vi "ProcAndStates.vi"(0 "spreadsheet string":string=" Инициализация\r\nНачало\r\nВосстановлениеУправления\r\nНачалоРаботы\r\n ОстановВсехПроцессовИстартПроцИнициализация\r\nНачало\r\n КонтрольДостоверности\r\nНачало\r\nОстановПроцессов\r\nСообК_ГУИ_НЕТ_ДОСТОВЕРНОСТИ\r\nНарушениеСвязи\r\n КонтрольДостоверностиОткрытияЗатвораВакуумного\r\nНачало\r\nСменаСостоянияВКЛ\r\nСменаСостоянияВЫКЛ\r\nТрафикПауза\r\nНарушениеСвязи\r\n КонтрольДостоверностиОткрЗатВакуумного\r\nНачало\r\nСообК_ГУИ_ЕСТЬ_ДОСТОВЕРНОСТЬ\r\nОжиданиеНедостоверности\r\nСообК_ГУИ_НЕТ_ДОСТОВЕРНОСТИ\r\nОжиданиеЕстьДостоверность\r\nНарушениеСвязи\r\n КонтрольДостоверностиЗакрЗатВакуумного\r\nНачало\r\nСообК_ГУИ_ЕСТЬ_ДОСТОВЕРНОСТЬ\r\nОжиданиеНедостоверности\r\nСообК_ГУИ_НЕТ_ДОСТОВЕРНОСТИ\r\nОжиданиеЕстьДостоверность\r\nНарушениеСвязи\r\n КонтрольДостоверностиСостоянияСапуна\r\nНачало\r\nСообК_ГУИ_ЕСТЬ_ДОСТОВЕРНОСТЬ\r\nОжиданиеНедостоверности\r\nСообК_ГУИ_НЕТ_ДОСТОВЕРНОСТИ\r\nОжиданиеЕстьДостоверность\r\nНарушениеСвязи\r\n КонтрольДостоверностиСостоянияУстройстваПлавПуска\r\nНачало\r\nСообК_ГУИ_ЕСТЬ_ДОСТОВЕРНОСТЬ\r\nОжиданиеНедостоверности\r\nСообК_ГУИ_НЕТ_ДОСТОВЕРНОСТИ\r\nОжиданиеЕстьДостоверность\r\nНарушениеСвязи\r\n КонтрольДостоверностиСостоянияПитанияВакуумногоНасоса\r\nНачало\r\nСообК_ГУИ_ЕСТЬ_ДОСТОВЕРНОСТЬ\r\nОжиданиеНедостоверности\r\nСообК_ГУИ_НЕТ_ДОСТОВЕРНОСТИ\r\nОжиданиеЕстьДостоверность\r\nНарушениеСвязи\r\n КонтрольДостоверностиСостоянияПитанияВентилятора\r\nНачало\r\nСообК_ГУИ_ЕСТЬ_ДОСТОВЕРНОСТЬ\r\nОжиданиеНедостоверности\r\nСообК_ГУИ_НЕТ_ДОСТОВЕРНОСТИ\r\nОжиданиеЕстьДостоверность\r\nНарушениеСвязи\r\n КонтрольДостоверностиСостоянияПитанияРегТемпературы\r\nНачало\r\nСообК_ГУИ_ЕСТЬ_ДОСТОВЕРНОСТЬ\r\nОжиданиеНедостоверности\r\nСообК_ГУИ_НЕТ_ДОСТОВЕРНОСТИ\r\nОжиданиеЕстьДостоверность\r\nНарушениеСвязи\r\n КонтрольДостоверностиСостоянияПитанияРегУровня\r\nНачало\r\nСообК_ГУИ_ЕСТЬ_ДОСТОВЕРНОСТЬ\r\nОжиданиеНедостоверности\r\nСообК_ГУИ_НЕТ_ДОСТОВЕРНОСТИ\r\nОжиданиеЕстьДостоверность\r\nНарушениеСвязи\r\n КонтрольДостоверностиУровняВодыМинимум\r\nНачало\r\nСообК_ГУИ_ЕСТЬ_ДОСТОВЕРНОСТЬ\r\nОжиданиеНедостоверности\r\nСообК_ГУИ_НЕТ_ДОСТОВЕРНОСТИ\r\nОжиданиеЕстьДостоверность\r\nНарушениеСвязи\r\n КонтрольДостоверностиУровняВодыМаксимум\r\nНачало\r\nСообК_ГУИ_ЕСТЬ_ДОСТОВЕРНОСТЬ\r\nОжиданиеНедостоверности\r\nСообК_ГУИ_НЕТ_ДОСТОВЕРНОСТИ\r\nОжиданиеЕстьДостоверность\r\nНарушениеСвязи\r\n КонтрольДостоверностиСостоянияПитанияНасОхлаждения\r\nНачало\r\nСообК_ГУИ_ЕСТЬ_ДОСТОВЕРНОСТЬ\r\nОжиданиеНедостоверности\r\nСообК_ГУИ_НЕТ_ДОСТОВЕРНОСТИ\r\nОжиданиеЕстьДостоверность\r\nНарушениеСвязи\r\n ЧтениеФактПараметров_с_Датчиков\r\nНачало\r\n РЕГУЛЯТОР_ТРАФИКА\r\nНачало\r\n ЧтениеКольцевогоБуфера\r\nНачало\r\nКонтрольВыполненияК\r\nКонтрольИзмененияНП\r\nНекорректноеСобытие\r\nНарушениеСвязи\r\n ОбработкаКомандИзмененияНП_от_ГУИ\r\nАнализ\r\nПодтверждениеИзмененияНП\r\nНекорректноеСобытие\r\nНарушениеСвязи\r\n ОбработкаКомандУправления_от_ГУИ\r\nАнализ\r\nНекорректноеСобытие\r\nПередачаСообщенияСПараметромГУИ\r\nНарушениеСвязи\r\n КонтрольИзменения_ФП_P_ВбакеКомпрессора\r\nНачало\r\nКонтрольИзменения\r\nСообщОбИзменении\r\nТрафикПауза\r\nНарушениеСвязи\r\n КонтрольИзменения_ФП_P_Впатрубке\r\nНачало\r\nКонтрольИзменения\r\nСообщОбИзменении\r\nТрафикПауза\r\nНарушениеСвязи\r\n КонтрольИзменения_ФП_T_Врубашке\r\nНачало\r\nКонтрольИзменения\r\nСообщОбИзменении\r\nТрафикПауза\r\nНарушениеСвязи\r\n КонтрольИзменения_ФП_T_Вбаке\r\nНачало\r\nКонтрольИзменения\r\nСообщОбИзменении\r\nТрафикПауза\r\nНарушениеСвязи\r\n КонтрольИзменения_ФП_P_ВтрубеСидер\r\nНачало\r\nКонтрольИзменения\r\nСообщОбИзменении\r\nТрафикПауза\r\nНарушениеСвязи\r\n КонтрольВеличиныОткачкиВауумнойТрубыСидеростата\r\nНачало\r\nАнализОткачки\r\n КонтрольГотовностиВакуума_в_Вакуумной_Трубе\r\nНачало\r\nДавлениеНормальное\r\nДавлениеВысокое\r\nЗадержка\r\nНарушениеСвязи\r\n КонтрольУровняВодыБакаОхлаждения\r\nНачало\r\nНизкийУровеньВоды\r\nВысокийУровеньВоды\r\nУровеньВодыВнорме\r\nЗадержка\r\nНарушениеСвязи\r\n КонтрольТемпературыВодыБакаОхлаждения\r\nНачало\r\nНизкаяТемператураВоды\r\nВысокаяТемператураВоды\r\nТемператураВнорме\r\nЗадержка\r\nНарушениеСвязи\r\n КонтрольТемпературыРубашкиОхлаждения\r\nНачало\r\nНизкаяТемператураВоды\r\nВысокаяТемператураВоды\r\nТемператураВнорме\r\nЗадержка\r\nНарушениеСвязи\r\n КонтрольДавленияВбакеКомпрессора\r\nНачало\r\nНизкоеДавление\r\nДавлениеВнорме\r\nЗадержка\r\nНарушениеСвязи\r\n ВКЛ_ПИТ_ВЕНТИЛЯТОР\r\nНачало\r\nКонтрольВключения\r\nПередачаСообщения\r\nОшибка\r\nНарушениеСвязи\r\n ВЫК_ПИТ_ВЕНТИЛЯТОР\r\nНачало\r\nКонтрольВыключения\r\nПередачаСообщения\r\nОшибка\r\nНарушениеСвязи\r\n КонтрольСостоянияПитанияВентилятора\r\nНачало\r\nСменаСостоянияВКЛ\r\nСменаСостоянияВЫКЛ\r\nНарушениеСвязи\r\n КонтрольСпонтанногоВыключенияВентилятора\r\nКонтроль\r\nОшибка\r\nНарушениеСвязи\r\n КонтрольСпонтанногоВключенияВентилятора\r\nКонтроль\r\nОшибка\r\nНарушениеСвязи\r\n КонтрольСостоянияЗатвораВакуумного\r\nНачало\r\nСменаСостоянияСреднего\r\nСменаСостоянияЗакрытия\r\nСменаСостоянияОткрытия\r\nСменаСостоянияОшибки\r\nНарушениеСвязи\r\n ОТКР_ЗАТВОР_ВАК\r\nНачало\r\nКонтроль\r\nПередачаСообщения\r\nОшибка\r\nНарушениеСвязи\r\n ЗАКР_ЗАТВОР_ВАК\r\nНачало\r\nКонтроль\r\nПередачаСообщения\r\nОшибка\r\nНарушениеСвязи\r\n КонтрольСпонтанногоЗакрытияЗатвораВакуумного\r\nКонтрольЗакрытия\r\nОшибка\r\nНарушениеСвязи\r\n КонтрольСпонтанногоОткрытияЗатвораВакуумного\r\nКонтроль\r\nОшибка\r\nНарушениеСвязи\r\n ОТКР_САПУН\r\nНачало\r\nКонтрольОткрытия\r\nПередачаСообщения\r\nОшибка\r\nНарушениеСвязи\r\n ЗАКР_САПУН\r\nНачало\r\nКонтрольЗакрытия\r\nПередачаСообщения\r\nОшибка\r\nНарушениеСвязи\r\n КонтрольСостоянияПитанияСапуна\r\nНачало\r\nСменаСостоянияВКЛ\r\nСменаСостоянияВЫКЛ\r\nНарушениеСвязи\r\n КонтрольСпонтанногоЗакрытияСапуна\r\nКонтрольЗакрытия\r\nОшибка\r\nНарушениеСвязи\r\n КонтрольСпонтанногоОткрытияСапуна\r\nКонтроль\r\nОшибка\r\nНарушениеСвязи\r\n ВКЛ_ПИТ_ВАК_НАСОСА\r\nНачало\r\nКонтрольВключения\r\nПередачаСообщения\r\nОшибка\r\nНарушениеСвязи\r\n ВЫК_ПИТ_ВАК_НАСОСА\r\nНачало\r\nКонтрольВыключения\r\nОшибка\r\nНарушениеСвязи\r\nПередачаСообщения\r\n КонтрольСостоянияПитанияВакуумногоНасоса\r\nНачало\r\nСменаСостоянияВКЛ\r\nСменаСостоянияВЫКЛ\r\nНарушениеСвязи\r\n КонтрольСпонтанногоВыключенияВакНасоса\r\nКонтроль\r\nОшибка\r\nНарушениеСвязи\r\n КонтрольСпонтанногоВключенияВакНасоса\r\nКонтроль\r\nОшибка\r\nНарушениеСвязи\r\n ВКЛ_ПИТ_РЕГ_Т\r\nНачало\r\nКонтрольВключения\r\nПередачаСообщения\r\nОшибка\r\nНарушениеСвязи\r\n ВЫК_ПИТ_РЕГ_Т\r\nНачало\r\nКонтрольВыключения\r\nПередачаСообщения\r\nОшибка\r\nНарушениеСвязи\r\n КонтрольСостоянияПитанияРЕГ_Т\r\nНачало\r\nСменаСостоянияВКЛ\r\nСменаСостоянияВЫКЛ\r\nНарушениеСвязи\r\n КонтрольСпонтанногоВыключенияРЕГ_Т\r\nКонтроль\r\nОшибка\r\nНарушениеСвязи\r\n КонтрольСпонтанногоВключенияРЕГ_Т\r\nКонтроль\r\nОшибка\r\nНарушениеСвязи\r\n ВКЛ_ПИТ_РЕГ_УР\r\nНачало\r\nКонтроль\r\nПередачаСообщения\r\nОшибка\r\nНарушениеСвязи\r\n ВЫК_ПИТ_РЕГ_УР\r\nНачало\r\nКонтроль\r\nПередачаСообщения\r\nОшибка\r\nНарушениеСвязи\r\n КонтрольСостоянияПитанияРЕГ_УР\r\nНачало\r\nСменаСостоянияВКЛ\r\nСменаСостоянияВЫКЛ\r\nНарушениеСвязи\r\n КонтрольСпонтанногоВыключенияРЕГ_УР\r\nКонтроль\r\nОшибка\r\nНарушениеСвязи\r\n КонтрольСпонтанногоВключенияРЕГ_УР\r\nКонтроль\r\nОшибка\r\nНарушениеСвязи\r\n ВКЛ_ПИТ_НАС_ОХЛ\r\nНачало\r\nВключениеПитания\r\nКонтроль\r\nПередачаСообщения\r\nОшибка\r\nНарушениеСвязи\r\n ВЫК_ПИТ_НАС_ОХЛ\r\nНачало\r\nКонтроль\r\nПередачаСообщения\r\nОшибка\r\nНарушениеСвязи\r\n КонтрольСостоянияПитанияНАС_ОХЛ\r\nНачало\r\nСменаСостоянияВКЛ\r\nСменаСостоянияВЫКЛ\r\nНарушениеСвязи\r\n КонтрольСпонтанногоВыключенияНасосаОхлаждения\r\nКонтроль\r\nОшибка\r\nНарушениеСвязи\r\n КонтрольСпонтанногоВключенияНасосаОхлаждения\r\nКонтроль\r\nОшибка\r\nНарушениеСвязи\r\n ВКЛ_УСТР_ПЛАВ_ПУСКА\r\nНачало\r\nКонтроль\r\nПередачаСообщения\r\nОшибка\r\nНарушениеСвязи\r\n ВЫК_УСТР_ПЛАВ_ПУСКА\r\nНачало\r\nКонтрольВыключения\r\nПередачаСообщения\r\nОшибка\r\nНарушениеСвязи\r\n КонтрольСостоянияПитанияПЛАВ_ПУСКА\r\nНачало\r\nСменаСостоянияВКЛ\r\nСменаСостоянияВЫКЛ\r\nНарушениеСвязи\r\n КонтрольСпонтанногоВыключенияПлавнПуска\r\nКонтроль\r\nОшибка\r\nНарушениеСвязи\r\n КонтрольСпонтанногоВключенияПлавнПуска\r\nКонтроль\r\nОшибка\r\nНарушениеСвязи\r\n ВКЛ_ВАКУУМИРОВАНИЕ_ТРУБЫ\r\nНачало\r\nПроверкаНеобходимостиВакуумирования\r\nПередачаСообщения\r\nКонтрольВключенияВакПодсистемы\r\nЗапоминаемДавлениеВвакуумнойТрубе\r\nКонтрольТемпературыРубашки\r\nКонтрольРаботыОборудования\r\nКонтрольДавления\r\nСообщениеОКонцеВакуумирования\r\nПаузаНаРазвакуумированиеТрубы\r\nПаузаНаОткачкуВвакуумнойТрубе\r\nПроверкаУменьшенияДавленияВпатрубке\r\nОткачкаОтсутствует\r\nВыключениеВакуумнойПодсистемы\r\nСообщениеОбОтказеВакуумирования\r\nНарушениеСвязи\r\n ВЫК_ВАКУУМИРОВАНИЕ_ТРУБЫ\r\nНачало\r\nПередачаСообщения\r\nВыключениеВакуумнойПодсистемы\r\nНарушениеСвязи\r\n ВКЛ_ВАКУУМНУЮ_ПОДСИСТЕМУ\r\nНачало\r\nВключениеПитанияРегУровня\r\nКонтрольВключенияПитРегУр\r\nКонтрольГотовностиУровняВодыБО\r\nВключениеРегТ\r\nКонтрольВключенияРегТ\r\nКонтрольПревышенияТемпературыВодыБО\r\nКонтрольГотовностиТемпературыВодыБО\r\nВключаемВентилятор\r\nКонтрольВключенияВентилятора\r\nКонтрольВключенияПитанияНасосаОхлаждения\r\nКонтрольЗакрытияЗатвораВакуумного\r\nКонтрольОткрытияСапуна\r\nКонтрольТемпературыРубашки\r\nПодачаПитанияНаВакуумныйНасос\r\nКонтрольПитанияВакуумногоНасоса\r\nВключениеУстройстваПлавногоПуска\r\nКонтрольВлюченияПлавногоПуска\r\nТаймаутПередЗакрытиемСапуна\r\nЗакрытиеСапуна\r\nКонтрольЗакрытияСапуна\r\nЗапоминаемДавлениеВпатрубке\r\nКонтрольДавления\r\nПаузаНаОткачкуВпатрубке\r\nПроверкаУменьшенияДавленияВпатрубке\r\nКонтрольОткрытияЗВ\r\nОшибка\r\nВыключениеПоОшибке\r\nСообщениеОбОтказеВакуумирования\r\nНарушениеСвязи\r\n ВЫК_ВАКУУМНУЮ_ПОДСИСТЕМУ\r\nНачало\r\nКонтрольЗакрытияЗатвораВакуумного\r\nКонтрольОткрытияСапуна\r\nТаймаутПередВыключениемПитанияВакуумногоНасоса\r\nВыключаемУППВакуумногоНасоса\r\nКонтрольВыключенияПитанияУППВакуумногоНасоса\r\nКонтрольВыключенияПитанияВакуумногоНасоса\r\nКонтрольВыключенияНасосаОхлаждения\r\nКонтрольВыключенияВентилятора\r\nСообщениеОбОтказеВыклВакСистемы\r\nНарушениеСвязи\r\n") -> (1 "PROCESSES":string[](array[string])=["Инициализация", "ОстановВсехПроцессовИстартПроцИнициализация", "КонтрольДостоверности", "КонтрольДостоверностиОткрытияЗатвораВакуумного", "КонтрольДостоверностиОткрЗатВакуумного", "КонтрольДостоверностиЗакрЗатВакуумного", "КонтрольДостоверностиСостоянияСапуна", "КонтрольДостоверностиСостоянияУстройстваПлавПуска", "КонтрольДостоверностиСостоянияПитанияВакуумногоНасоса", "КонтрольДостоверностиСостоянияПитанияВентилятора", "КонтрольДостоверностиСостоянияПитанияРегТемпературы", "КонтрольДостоверностиСостоянияПитанияРегУровня", "КонтрольДостоверностиУровняВодыМинимум", "КонтрольДостоверностиУровняВодыМаксимум", "КонтрольДостоверностиСостоянияПитанияНасОхлаждения", "ЧтениеФактПараметров_с_Датчиков", "РЕГУЛЯТОР_ТРАФИКА", "ЧтениеКольцевогоБуфера", "ОбработкаКомандИзмененияНП_от_ГУИ", "ОбработкаКомандУправления_от_ГУИ", "КонтрольИзменения_ФП_P_ВбакеКомпрессора", "КонтрольИзменения_ФП_P_Впатрубке", "КонтрольИзменения_ФП_T_Врубашке", "КонтрольИзменения_ФП_T_Вбаке", "КонтрольИзменения_ФП_P_ВтрубеСидер", "КонтрольВеличиныОткачкиВауумнойТрубыСидеростата", "КонтрольГотовностиВакуума_в_Вакуумной_Трубе", "КонтрольУровняВодыБакаОхлаждения", "КонтрольТемпературыВодыБакаОхлаждения", "КонтрольТемпературыРубашкиОхлаждения", "КонтрольДавленияВбакеКомпрессора", "ВКЛ_ПИТ_ВЕНТИЛЯТОР", "ВЫК_ПИТ_ВЕНТИЛЯТОР", "КонтрольСостоянияПитанияВентилятора", "КонтрольСпонтанногоВыключенияВентилятора", "КонтрольСпонтанногоВключенияВентилятора", "КонтрольСостоянияЗатвораВакуумного", "ОТКР_ЗАТВОР_ВАК", "ЗАКР_ЗАТВОР_ВАК", "КонтрольСпонтанногоЗакрытияЗатвораВакуумного", "КонтрольСпонтанногоОткрытияЗатвораВакуумного", "ОТКР_САПУН", "ЗАКР_САПУН", "КонтрольСостоянияПитанияСапуна", "КонтрольСпонтанногоЗакрытияСапуна", "КонтрольСпонтанногоОткрытияСапуна", "ВКЛ_ПИТ_ВАК_НАСОСА", "ВЫК_ПИТ_ВАК_НАСОСА", "КонтрольСостоянияПитанияВакуумногоНасоса", "КонтрольСпонтанногоВыключенияВакНасоса", "КонтрольСпонтанногоВключенияВакНасоса", "ВКЛ_ПИТ_РЕГ_Т", "ВЫК_ПИТ_РЕГ_Т", "КонтрольСостоянияПитанияРЕГ_Т", "КонтрольСпонтанногоВыключенияРЕГ_Т", "КонтрольСпонтанногоВключенияРЕГ_Т", "ВКЛ_ПИТ_РЕГ_УР", "ВЫК_ПИТ_РЕГ_УР", "КонтрольСостоянияПитанияРЕГ_УР", "КонтрольСпонтанногоВыключенияРЕГ_УР", "КонтрольСпонтанногоВключенияРЕГ_УР", "ВКЛ_ПИТ_НАС_ОХЛ", "ВЫК_ПИТ_НАС_ОХЛ", "КонтрольСостоянияПитанияНАС_ОХЛ", "КонтрольСпонтанногоВыключенияНасосаОхлаждения", "КонтрольСпонтанногоВключенияНасосаОхлаждения", "ВКЛ_УСТР_ПЛАВ_ПУСКА", "ВЫК_УСТР_ПЛАВ_ПУСКА", "КонтрольСостоянияПитанияПЛАВ_ПУСКА", "КонтрольСпонтанногоВыключенияПлавнПуска", "КонтрольСпонтанногоВключенияПлавнПуска", "ВКЛ_ВАКУУМИРОВАНИЕ_ТРУБЫ", "ВЫК_ВАКУУМИРОВАНИЕ_ТРУБЫ", "ВКЛ_ВАКУУМНУЮ_ПОДСИСТЕМУ", "ВЫК_ВАКУУМНУЮ_ПОДСИСТЕМУ"], 2 "STATES":string[][](array[string]))   [LabVIEW 2012]
panel:
  out "size(s)":i32[](array[numeric])=[75, 0]
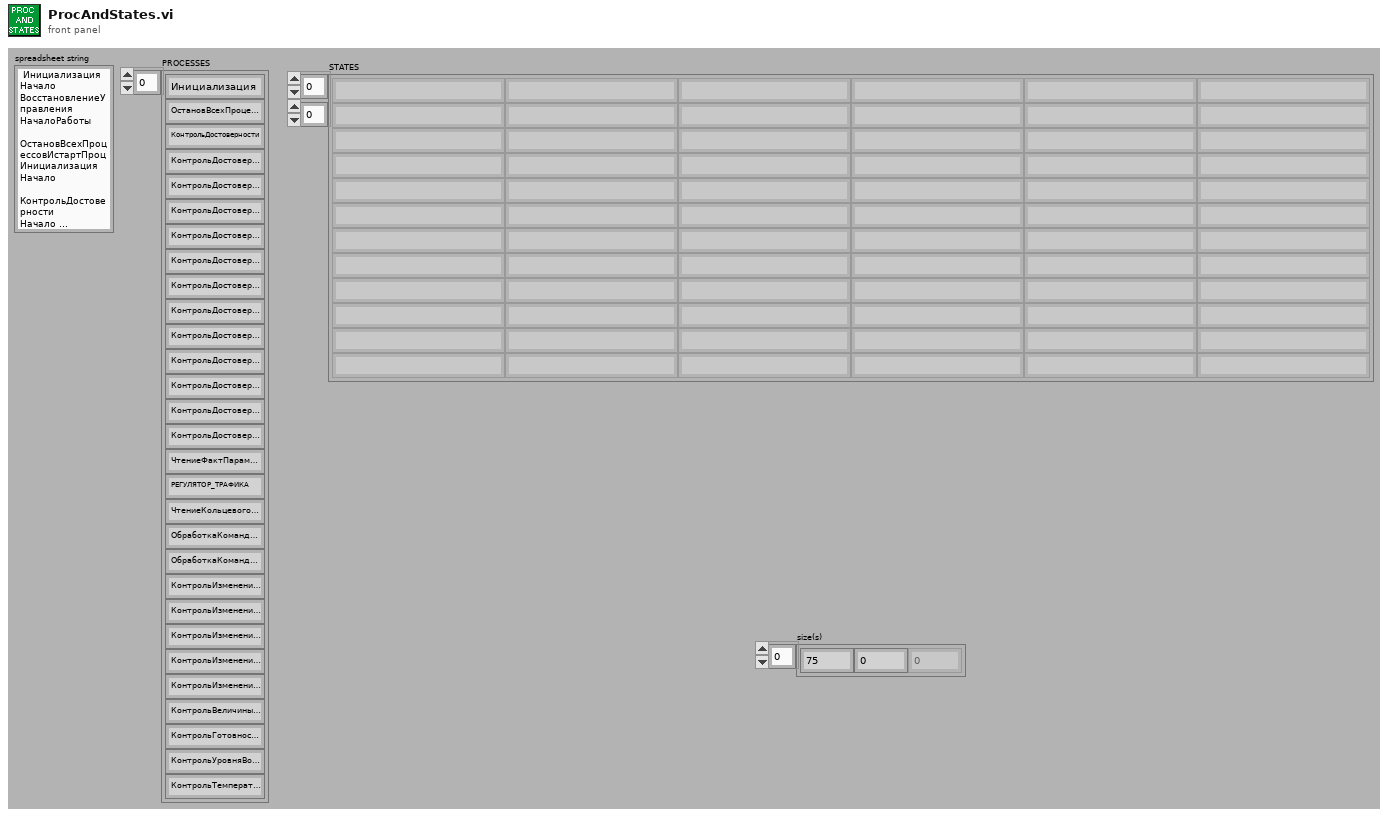
[diagram p1: front panel]
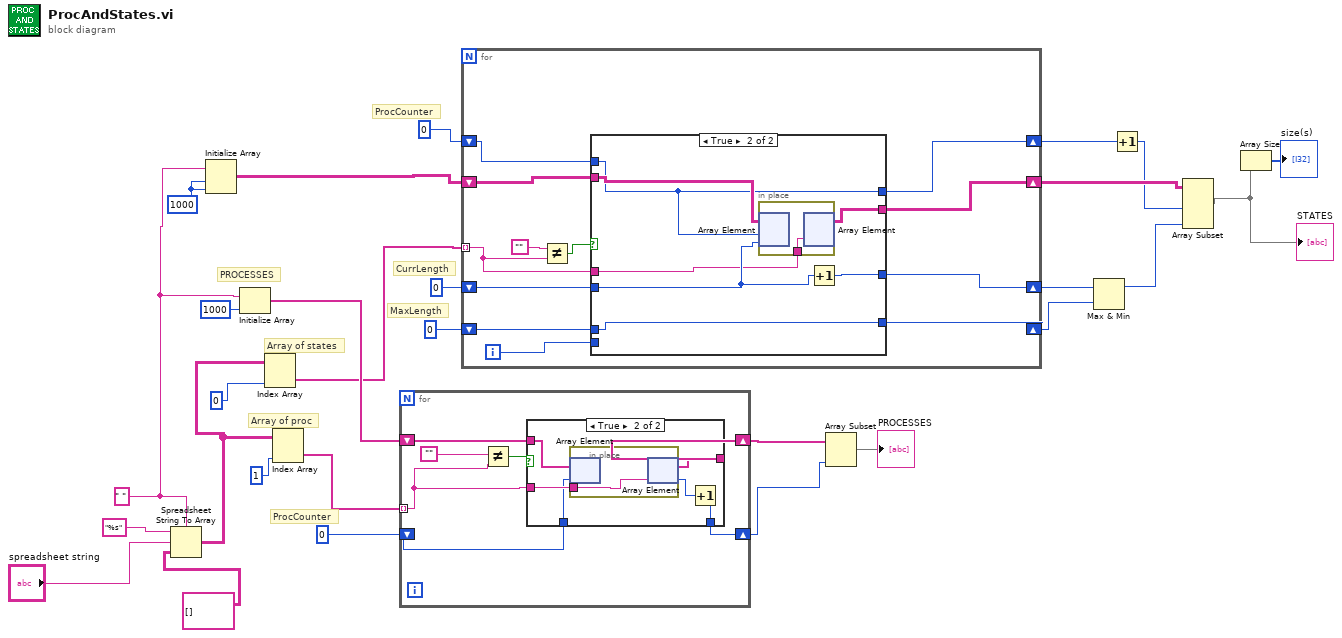
[diagram p0: block diagram]
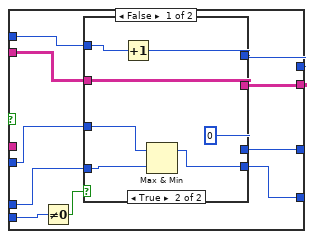
[diagram p2: hidden frame]
diagram:
  w15 = 1000 ("dimension size")
  w16 = " " ("delimiter (Tab)")
  # "ProcCounter"
  # "PROCESSES"
  # "CurrLength"
  # "MaxLength"
  # "ProcCounter"
  # "Array of proc"
  # "Array of states"
  n1 = Spreadsheet String To Array(delimiter (Tab)=w16, format string="%s", spreadsheet string="spreadsheet string", array type (2D Dbl)=string[][] []) -> (array=w27:string[][])
  n2 = Initialize Array(w16, w15, w15) -> (w20:string[][])
  n3 = Initialize Array(w16, 1000 ("dimension size")) -> (w23:string[])
  n4 = Index Array(array=w27, index (col)=0 ("index (row)")) -> (element=w17:string[])  [unwired: 1 in]
  n5 = Index Array(array=w27, index (col)=1 ("index (row)")) -> (element=w22:string[])  [unwired: 1 in]
  n6 = for {
    tunnel: w22 -> [w34] mode=indexing
    shift-right: [w32] -> w9
    shift-left: w23 -> [w33]
    shift-right: [w29] -> w6
    shift-left: 0 ("dimension size") -> [w30]
    n7 = Not Equal?(x="", y=w34) -> (x != y?=w35:bool)
    n8 = case shown="True" w35 {
      tunnel: w34 -> [_ w42]
      tunnel: w33 -> [w37 w43]
      tunnel: [w37 w38] -> w32
      tunnel: w30 -> [w36 w41]
      tunnel: [w36 w39] -> w29
      frame False {
      }
      frame True {
        n9 = in-place {
          in-place-border: w42 -> [w44]
          n10 = in-place-array #1(w43, w41) -> ()  [unwired: 1 out]
          n11 = in-place-array #1(w44) -> (w38:string[], w40:i32)
        }
        n12 = Increment(x=w40) -> (x+1=w39:i32)
      }
    }
  }
  n13 = for {
    tunnel: w17 -> [w54] mode=indexing
    shift-right: [w50] -> w2
    shift-left: w20 -> [w55]
    shift-right: [w52] -> w13
    shift-left: 0 ("dimension size") -> [w53]
    shift-right: [w49] -> w11
    shift-left: 0 ("dimension size") -> [w51]
    shift-right: [w45] -> w12
    shift-left: 0 ("dimension size") -> [w46]
    i -> [w47]
    n14 = Not Equal?(x="", y=w54) -> (x != y?=w56:bool)
    n15 = case shown="True" w56 {
      tunnel: [w65 w81] -> w50
      tunnel: w55 -> [w66 w82]
      tunnel: w54 -> [_ w79]
      tunnel: w53 -> [w64 w78]
      tunnel: [w57 w78] -> w52
      tunnel: w51 -> [w63 w84]
      tunnel: [w62 w84] -> w49
      tunnel: w47 -> [w61 _]
      tunnel: w46 -> [w59 w80]
      tunnel: [w58 w83] -> w45
      frame False {
        n16 = Not Equal To 0?(x=w61) -> (x != 0?=w60:bool)
        n17 = case shown="True" w60 {
          tunnel: w66 -> [w70 w73]
          tunnel: [w70 w73] -> w65
          tunnel: w64 -> [w68 w77]
          tunnel: [w68 w72] -> w57
          tunnel: w63 -> [w69 w76]
          tunnel: [w69 w71] -> w62
          tunnel: w59 -> [w67 w75]
          tunnel: [w67 0] -> w58
          frame False {
          }
          frame True {
            n18 = Increment(x=w77) -> (x+1=w72:i32)
            n19 = Max & Min(x=w75, y=w76) -> (max(x,y)=w71:i32)  [unwired: 1 out]
          }
        }
      }
      frame True {
        n20 = in-place {
          in-place-border: w79 -> [w85]
          n21 = in-place-array #2(w82, w78, w80) -> ()  [unwired: 1 out]
          n22 = in-place-array #2(w85) -> (w81:string[][])  [unwired: 2 out]
        }
        n23 = Increment(x=w80) -> (x+1=w83:i32)
      }
    }
  }
  n24 = Array Subset(array=w9, length=w6) -> (→"PROCESSES":string[])  [unwired: 1 in]
  n25 = Max & Min(x=w12, y=w11) -> (max(x,y)=w5:i32)  [unwired: 1 out]
  n26 = Increment(x=w13) -> (x+1=w1:i32)
  n27 = Array Subset(array=w2, length (row)=w1, length (col)=w5) -> (w4:string[][])  [unwired: 2 in]
  "STATES" <- w4
  n28 = Array Size(array=w4) -> (size(s)=→"size(s)":i32[])
